vi "Map Tags to Channels.vi"(7 "instance id":string, 8 "error in (no error)":errorcluster, 9 "String Array":string[](array[string]), 10 "Lines":T1[](array[typedef]), 11 "engine configuration in":refnum<class "engine configuration.lvclass">) -> (0 "error out":errorcluster, 3 "engine configuration out":refnum<class "engine configuration.lvclass">)   [LabVIEW 2017, in "J1939 editor node.lvclass"]
uses:
  J1939 editor node.lvclass
  <vilib>/NI/Module Execution Interface/Engine Configuration/engine configuration.lvclass
  module/configuration/Line.ctl
  <vilib>/NI/Tag Bus Module Framework/channel/TBM channel.lvclass
  C:/Program Files (x86)/National Instruments/LabVIEW 2017/vi.lib/NI/Tag Bus/tag/tag descriptor.lvclass
  <vilib>/NI/Tag Bus/tag/tag descriptor.lvclass/tag descriptor.ctl
  <vilib>/NI/Tag Bus/tag/tag descriptor.lvclass
  module/configuration/J1939 configuration.lvclass
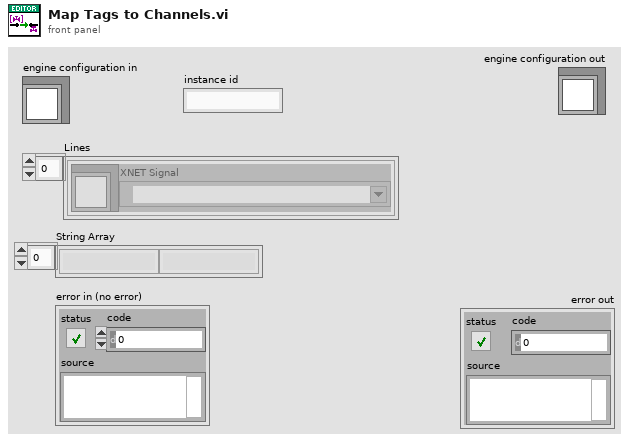
[diagram p1: front panel]
types:
  T1 = typedef "J1939 configuration.lvclass/Line.ctl" = cluster{"channel":refnum<class "TBM channel.lvclass">, "XNET Signal":refnum<k21>}
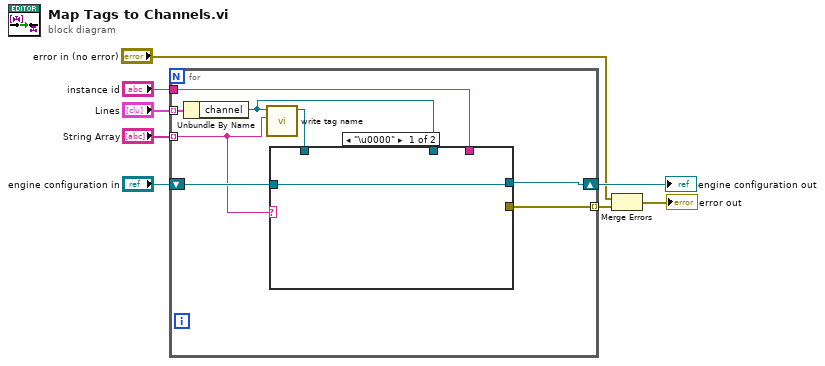
[diagram p0: block diagram]
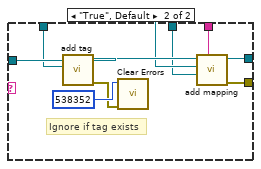
[diagram p2: hidden frame]
diagram:
  n1 = for {
    shift-right: [w16] -> w4
    shift-left: "engine configuration in" -> [w13]
    tunnel: "instance id" -> [w15]
    tunnel: "Lines" -> [w14] mode=indexing
    tunnel: "String Array" -> [w9] mode=indexing
    tunnel: [w11] -> w3 mode=indexing
    n2 = Unbundle By Name(w14) -> ("channel"=w10:refnum<class "TBM channel.lvclass">)
    n3 = call <vilib>:"write tag name.vi"("name"=w9, "system tag in"=w10) -> ("system tag out"=w12:refnum<class "TBM channel.lvclass">)  [unwired: 8 in, 1 out]
    n4 = case shown="\"\"" w9 {
      tunnel: [w17 w26] -> w16
      tunnel: w15 -> [_ w25]
      tunnel: w13 -> [w17 w23]
      tunnel: w12 -> [_ w20]
      tunnel: [_ w19] -> w11
      tunnel: w10 -> [_ w18]
      frame "\u0000" {
      }
      frame "True", Default {
        # "Ignore if tag exists"
        n5 = call-dynamic "add tag.vi"("tag descriptor"=w20, "engine configuration in"=w23) -> ("error out"=w22:errorcluster, "engine configuration out"=w21:refnum<class "engine configuration.lvclass">)  [unwired: 8 in]
        n6 = call <vilib>:"Clear Errors.vi"("error in (no error)"=w22, "specific error code to clear (0: all)"=538352) -> ()  [unwired: 4 in, 2 out]
        n7 = call-dynamic "add mapping.vi"("owner ID"=w25, "channel"=w18, "tag descriptor"=w20, "engine configuration"=w21) -> ("error out"=w19:errorcluster, "engine configuration out"=w26:refnum<class "engine configuration.lvclass">)  [unwired: 6 in]
      }
    }
  }
  "engine configuration out" <- w4
  n8 = Merge Errors("error in (no error)", w3) -> (→"error out":errorcluster)
